vi "YOLOv9_OpenVINO_IR.vi"() -> ()   [LabVIEW 2018]
doc: "YOLOv9_OpenVINO_IR: This example is an object detection example of the YOLOv9 algorithm, which can perform object detection on real-time images captured by cameras IR is OpenVINO's proprietary optimized format model."
uses:
  vi.lib/VIRobotics/ModelZoo/Object_Detection/yolov8_openvino/InitialModel_yolov9_OpenVINO_IR.vi
  vi.lib/VIRobotics/ModelZoo/Object_Detection/yolov8_openvino/yolov8_openvino.lvclass
  vi.lib/VIRobotics/opencv_yiku/Mat/Mat_8U/Mat_8U.lvclass
  vi.lib/VIRobotics/opencv_yiku/Cap/Cap.lvclass
panel:
  in  "device_name":string(combo)="CPU"
  in  "bin_fle":path
  out "每帧耗时(s)":dbl
  in  "class_names_file":path=path "C:/ProgramData/VIRobotics/ModelZoo/Object_Detection/coco.names"
  in  "xml file":path
  in  "stop":bool
  out "picture":picture
  # "Overview: Demonstrates how to use OpenVINO to load the the IR model of yolov9 for real-time object detection.\nRequirements: Windows.\nMake sure your computer has a camera。\nInstructions: \n1.Select the device_name to use.（If your computer has Intel GPU, you can select GPU in the \"type\" control before running the VI to achieve faster inference).\n2.Specify the xml_file、bin_file and class_names_file(Because the model is too large, it is not loaded by default.)\n3.Run the VI."
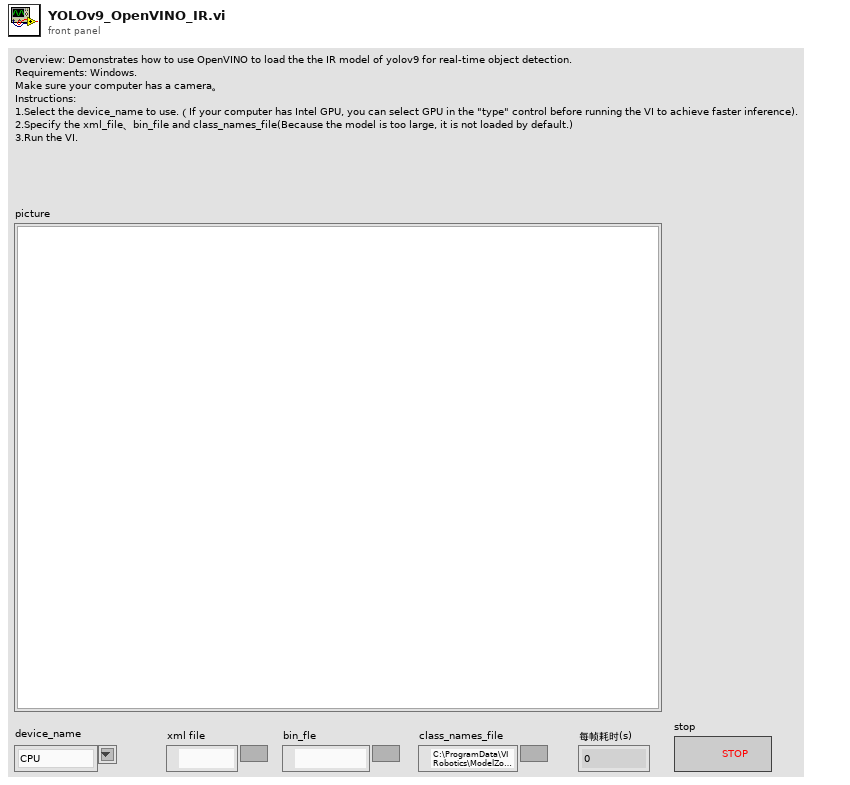
[diagram p1: front panel]
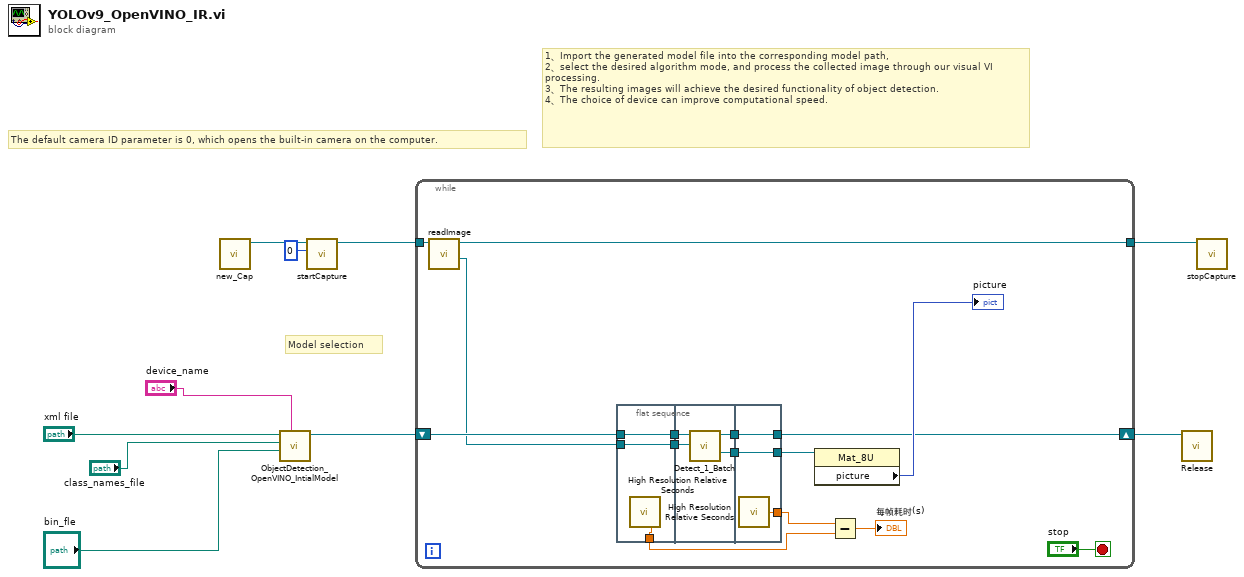
[diagram p0: block diagram]
diagram:
  # "1、Import the generated model file into the corresponding model path, \n2、select the desired algorithm mode, and process the collected image through our visual VI processing. \n3、The resulting images will achieve the desired functionality of object detection. \n4、The choice of device can improve computational speed."
  # "Model selection"
  # "The default camera ID parameter is 0, which opens the built-in camera on the computer."
  n1 = call "new_Cap.vi"() -> ("Cap out"=w10:refnum<class "Cap.lvclass">)  [unwired: 10 in, 1 out]
  n2 = call-poly "ObjectDetection_OpenVINO_IntialModel.vi"("device_name"="device_name", "bin_fle"="bin_fle", "class_names_path"="class_names_file", "xmlPath"="xml file") -> ("yolov9_openvino out"=w5:refnum<class "yolov8_openvino.lvclass">)  [unwired: 6 in, 1 out]
  n3 = call "startCapture.vi"("cameraID"=0, "Cap in"=w10) -> ("Cap out"=w8:refnum<class "Cap.lvclass">)  [unwired: 8 in, 1 out]
  n4 = while {
    tunnel: w8 -> [w24]
    shift-right: [w20] -> w6
    shift-left: w5 -> [w25]
    tunnel: [w19] -> w7
    stop <- "stop" stop-if-true
    n5 = call "readImage.vi"("Cap in"=w24) -> ("Mat out"=w12:refnum<class "Mat_8U.lvclass">, "Cap out"=w19:refnum<class "Cap.lvclass">)  [unwired: 8 in, 1 out]
    n6 = flat-sequence {
      tunnel: w25 -> [w28]
      tunnel: [w28] -> w18
      tunnel: [w27] -> w14
      tunnel: w12 -> [w26]
      tunnel: [w26] -> w11
      tunnel: w18 -> [w32]
      tunnel: [w31] -> w17
      tunnel: [w30] -> w16
      tunnel: w11 -> [w29]
      tunnel: [w34] -> w20
      tunnel: [w35] -> w23
      tunnel: w17 -> [w35]
      tunnel: w16 -> [w34]
      tunnel: [w33] -> w15
      frame #0 {
        n7 = call <vilib>:"High Resolution Relative Seconds.vi"() -> ("relative seconds"=w27:dbl)
      }
      frame #1 {
        n8 = call-dynamic "Detect_1_Batch.vi"("image"=w29, "yolov8_openvino in"=w32) -> ("img out"=w31:refnum<class "Mat_8U.lvclass">, "yolov8_openvino out"=w30:refnum<class "yolov8_openvino.lvclass">)  [unwired: 6 in, 2 out]
      }
      frame #2 {
        n9 = call <vilib>:"High Resolution Relative Seconds.vi"() -> ("relative seconds"=w33:dbl)
      }
    }
    n10 = property class="Mat_8U"(reference=w23) -> ("picture"=→"picture":picture)  [unwired: 1 in, 2 out]
    n11 = Subtract(x=w15, y=w14) -> (x-y=→"每帧耗时(s)":dbl)
  }
  n12 = call-dynamic "Release.vi"("yolov8_openvino in"=w6) -> ()  [unwired: 9 in, 2 out]
  n13 = call "stopCapture.vi"("Cap in"=w7) -> ()  [unwired: 10 in, 1 out]
